vi "Get Aperture Time Info [DT] Core.vi"(8 "error in (no error)":errorcluster, 11 "CS++DMM in":refnum<class "CS++DMM.lvclass">) -> (0 "error out":errorcluster, 1 "aperture time units":i32, 2 "aperture time (sec)":dbl format="%^.2e", 3 "CS++DMM out":refnum<class "CS++DMM.lvclass">)   [LabVIEW 2013, in "CS++DMM.lvlib" / "CS++DMM.lvclass"]
doc: "This VI returns additional information about the state of the instrument. Specifically, it returns the aperture time and the aperture time units.\n\nNote: \n\n(1) This VI is part of the IviDmmDeviceInfo [DI] extension group."
uses:
  CS++DMM.lvclass
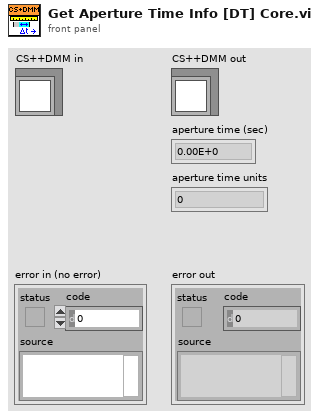
[diagram p1: front panel]
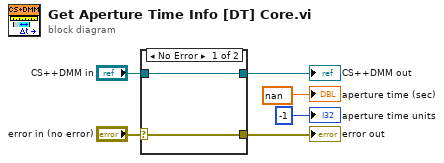
[diagram p0: block diagram]
diagram:
  n1 = case shown="No Error" "error in (no error)" {
    selector: "error in (no error)" -> [w7 w10]
    tunnel: [w7 w10] -> w5
    tunnel: [w8 w9] -> w3
    tunnel: "CS++DMM in" -> [w8 w9]
    frame No Error {
    }
    frame Error {
    }
  }
  "error out" <- w5
  "CS++DMM out" <- w3
  "aperture time (sec)" <- nan ("aperture time (sec)")
  "aperture time units" <- -1 ("aperture time units")
